vi "Show Waveform and XY Plots.vi"(3 "stop":bool, 4 "xy plot":picture, 5 "waveform plot":picture) -> ()   [LabVIEW 2010]
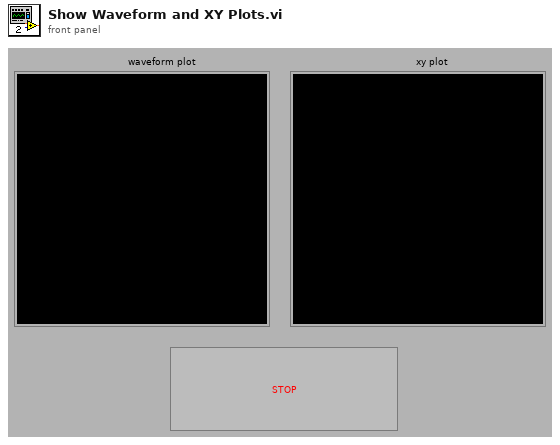
[diagram p1: front panel]
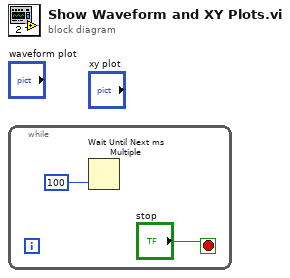
[diagram p0: block diagram]
diagram:
  n1 = while {
    stop <- "stop" stop-if-true
    n2 = Wait Until Next ms Multiple(millisecond multiple=u32 100) -> ()  [unwired: 1 out]
  }
